vi "share error upstream.vi"(10 "Error Object":refnum<class>, 11 "Template in":refnum<class "Template.lvclass">) -> ()   [LabVIEW 2020, in "Template.lvlib" / "Template.lvclass"]
doc: "Enqueues the call for generate an error event in the caller's enqueue."
uses:
  Template.lvclass
  C:/Program Files/National Instruments/LabVIEW 2020/vi.lib/ActorFramework/Actor/Actor.lvclass
  <vilib>/ActorFramework/Actor/Actor.lvclass/Actor.ctl
  <vilib>/ActorFramework/Message Enqueuer/Message Priority.ctl
  Template Messages/fire error object Msg/fire error object Msg.lvclass/fire error object Msg.ctl
  <vilib>/ActorFramework/Message Enqueuer/Message Enqueuer.lvclass/Message Enqueuer.ctl
  <vilib>/ActorFramework/Message Enqueuer/Enqueue.vi
  Template Messages/fire error object Msg/fire error object Msg.lvclass
  C:/Program Files/National Instruments/LabVIEW 2020/vi.lib/ActorFramework/Message/Message.lvclass
  <vilib>/ActorFramework/Message Priority Queue/Priority Enqueue.vi
  <vilib>/ActorFramework/Actor/Actor.lvclass
  <vilib>/ActorFramework/Message Enqueuer/Message Enqueuer.lvclass
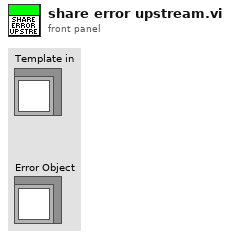
[diagram p1: front panel]
types:
  T1 = typedef "Actor Framework.lvlib/Message Enqueuer.lvclass/Message Priority.ctl" = enum16{"Low", "Normal", "High"}
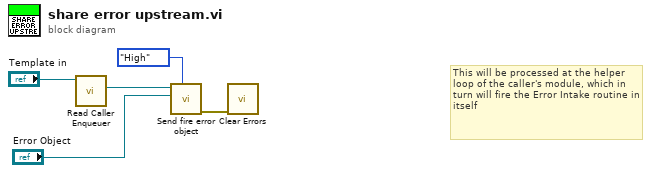
[diagram p0: block diagram]
diagram:
  # "This will be processed at the helper loop of the caller's module, which in turn will fire the Error Intake routine in itself"
  n1 = call <vilib>:"Read Caller Enqueuer.vi"("Actor"="Template in") -> ("Caller Enqueuer"=w4:refnum<class "Message Enqueuer.lvclass">)  [unwired: 10 in]
  n2 = call "Send fire error object.vi"("Message Priority (Normal)"=Message_Priority."High", "Error in"="Error Object", "Message Enqueuer"=w4) -> ("error out"=w1:errorcluster)  [unwired: 7 in, 1 out]
  n3 = call <vilib>:"Clear Errors.vi"("error in (no error)"=w1) -> ()  [unwired: 5 in, 2 out]
